vi "REM IO - Get Slave IOVars.vi"(8 "error in (no error)":errorcluster, 11 "ECAT Slave in":refnum<k21>="ni.var.io://localhost/EtherCAT Master/Device") -> (0 "error IO":errorcluster, 1 "REM IO Modules":refnum<k21>[](array[refnum]), 2 "ECAT Variablenobjekt":refnum<k21>[](array[refnum]), 3 "ECAT Slave out":refnum<k21>="ni.var.io:/")   [LabVIEW 2019, in "Scan Engine Custom Device.lvlib"]
uses:
  Scan Engine Custom Device.lvlib
  <resource>/objmgr/IndComECAT.rc
  <vilib>/NI VeriStand/Custom Device Tools/Custom Device Utility Library/Custom Device Utility Library.lvlib
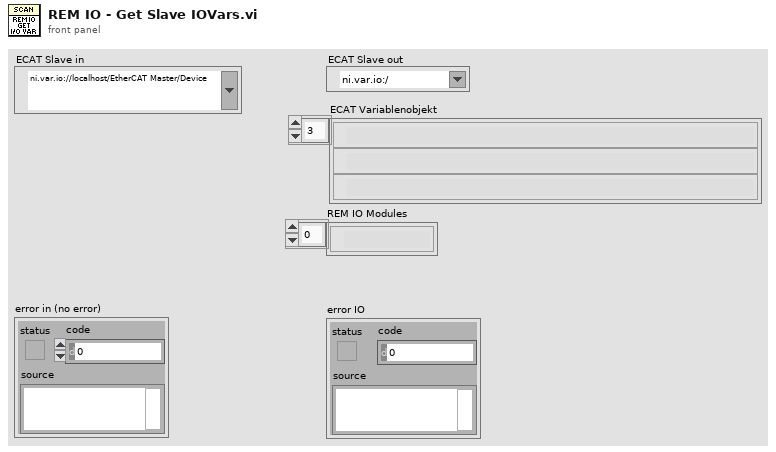
[diagram p1: front panel]
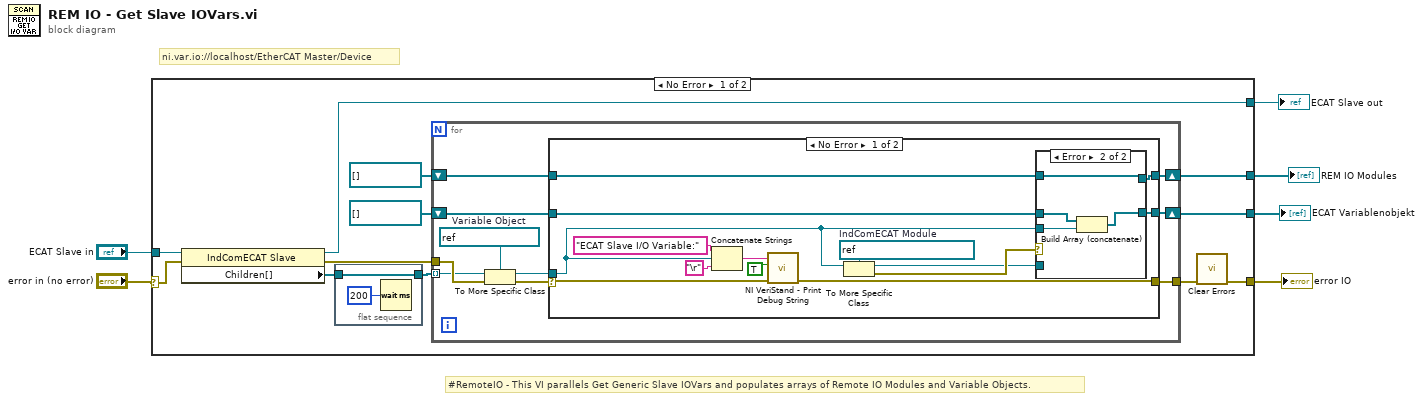
[diagram p0: block diagram]
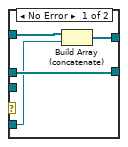
[diagram p2: hidden frame]
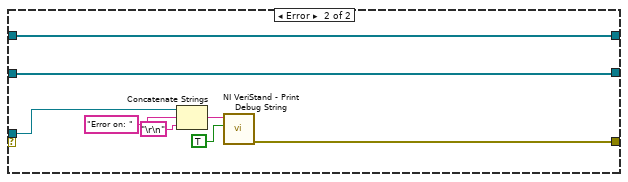
[diagram p3: hidden frame]
diagram:
  # "#RemoteIO - This VI parallels Get Generic Slave IOVars and populates arrays of Remote IO Modules and Variable Objects."
  # "ni.var.io://localhost/EtherCAT Master/Device"
  n1 = case shown="No Error" "error in (no error)" {
    selector: "error in (no error)" -> [w16 w62]
    tunnel: [w7 w62] -> w2
    tunnel: "ECAT Slave in" -> [w18 w61]
    tunnel: [w17 w61] -> w5
    tunnel: [w10 _] -> w3
    tunnel: [w8 _] -> w1
    frame No Error {
      n2 = property class="IndComECAT Slave"(reference=w18, error in=w16) -> (reference out=w17:refnum<k21>, error out=w15:errorcluster, "Children[]"=w13:refnum<k21>[])
      n3 = flat-sequence {
        tunnel: w13 -> [w20]
        tunnel: [w20] -> w12
        frame #0 {
          n4 = Wait (ms)(milliseconds to wait=u32 200) -> ()  [unwired: 1 out]
        }
      }
      n5 = for {
        tunnel: w12 -> [w26] mode=indexing
        tunnel: w15 -> [w30]
        tunnel: [w29] -> w14
        shift-right: [w25] -> w10
        shift-left: refnum<k21>[] [] -> [w24]
        shift-right: [w21] -> w8
        shift-left: refnum<k21>[] [] -> [w22]
        w23 = refnum<k21> refnum  # Variable Object
        n6 = To More Specific Class(target class=w23, reference=w26, error in=w30) -> (specific class reference=w27:refnum<k21>, error out=w28:errorcluster)
        n7 = case shown="No Error" w28 {
          selector: w28 -> [w40 _]
          tunnel: w27 -> [w35 w59]
          tunnel: [w41 w55] -> w29
          tunnel: [w43 w60] -> w25
          tunnel: w24 -> [w44 w60]
          tunnel: w22 -> [w33 w53]
          tunnel: [w32 w53] -> w21
          frame No Error {
            w36 = refnum<k21> refnum  # IndComECAT Module
            n8 = Concatenate Strings("ECAT Slave I/O Variable:", w35, "\r") -> (w39:string)
            n9 = call <vilib>:"NI VeriStand - Print Debug String.vi"("error in (no error)"=w40, "Add to log file? (F)"=TRUE, "Message"=w39) -> ("error out"=w41:errorcluster)  [unwired: 8 in]
            n10 = To More Specific Class(target class=w36, reference=w35) -> (specific class reference=w31:refnum<k21>, error out=w34:errorcluster)  [unwired: 1 in]
            n11 = case shown="Error" w34 {
              tunnel: w44 -> [w46 w52]
              tunnel: [w46 w50] -> w43
              tunnel: w35 -> [_ w51]
              tunnel: w33 -> [w48 w49]
              tunnel: [w47 w49] -> w32
              tunnel: w31 -> [w45 _]
              frame No Error {
                n12 = Build Array (concatenate)(w48, w45) -> (w47:refnum<k21>[])
              }
              frame Error {
                n13 = Build Array (concatenate)(w52, w51) -> (w50:refnum<k21>[])
              }
            }
          }
          frame Error {
            n14 = Concatenate Strings(w59, "Error on: ", "\r\n") -> (w56:string)
            n15 = call <vilib>:"NI VeriStand - Print Debug String.vi"("Add to log file? (F)"=TRUE ("Add to log file? (T)"), "Message"=w56) -> ("error out"=w55:errorcluster)  [unwired: 9 in]
          }
        }
      }
      n16 = call <vilib>:"Clear Errors.vi"("error in (no error)"=w14) -> ("error out"=w7:errorcluster)  [unwired: 5 in, 1 out]
    }
    frame Error {
    }
  }
  "error IO" <- w2
  "ECAT Slave out" <- w5
  "ECAT Variablenobjekt" <- w3
  "REM IO Modules" <- w1
